vi "solar_gbl Read Config.vi"(8 "error in (no error)":errorcluster, 10 "Name in":string, 11 "SOLAR in":T1) -> (0 "error out":errorcluster, 1 "Targets":string[][](array[string]), 2 "Name out":string, 3 "SOLAR out":T1)   [LabVIEW 2018]
doc: "This loads the default application settings from the solar.ini configuration file. The 'AppSetups' define the different application configuration sections that can override any default configuration keys. If the override key is not defined, this uses the default SOLAR applications settings. By default, the directories are located relative to the application executable."
uses:
  solar_ctl SOLAR Global.ctl
  solar_ctl Target Global.ctl
  voyager/solar_voy_ctl Voyager Refnum.ctl
  qtimer/solar_qtimer_ctl Refnum.ctl
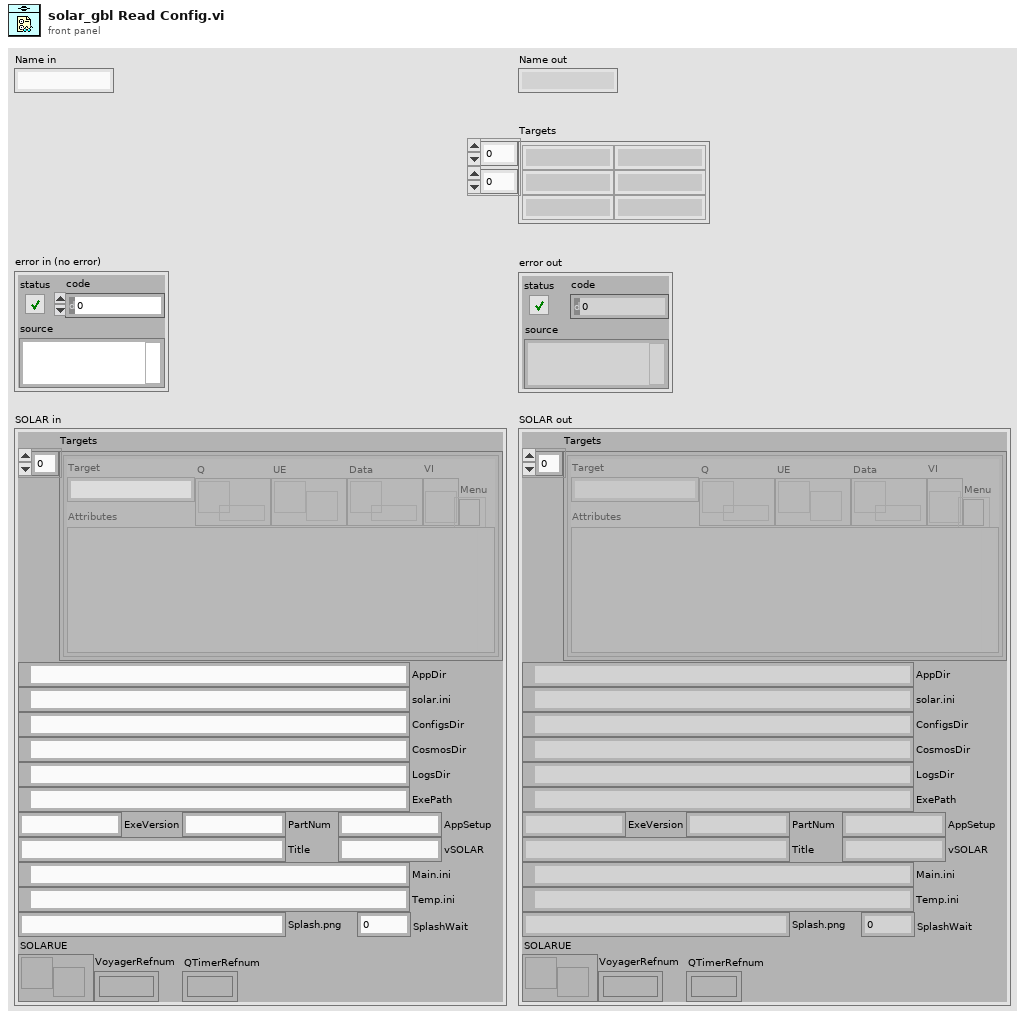
[diagram p1: front panel]
types:
  T1 = typedef "solar_ctl SOLAR Global.ctl" = cluster{"Targets":T2[], "AppDir":path, "solar.ini":path, "ConfigsDir":path, "CosmosDir":path, "LogsDir":path, "ExePath":path, "ExeVersion":string, "PartNum":string, "AppSetup":string, "Title":string, "Main.ini":path, "Temp.ini":path, "vSOLAR":string, "Splash.png":string, "SplashWait":i32, "SOLARUE":refnum<user-event>, "VoyagerRefnum":T3, "QTimerRefnum":T4}
  T2 = typedef "solar_ctl Target Global.ctl" = cluster{"Target":string, "Q":refnum<queue>, "UE":refnum<user-event>, "VI":refnum<vi>, "Menu":refnum<k9>, "Data":refnum<data-value>, "Attributes":variant}
  T3 = typedef "solar_voy_ctl Voyager Refnum.ctl" = refnum<k1>
  T4 = typedef "solar_qtimer_ctl Refnum.ctl" = refnum<k1>
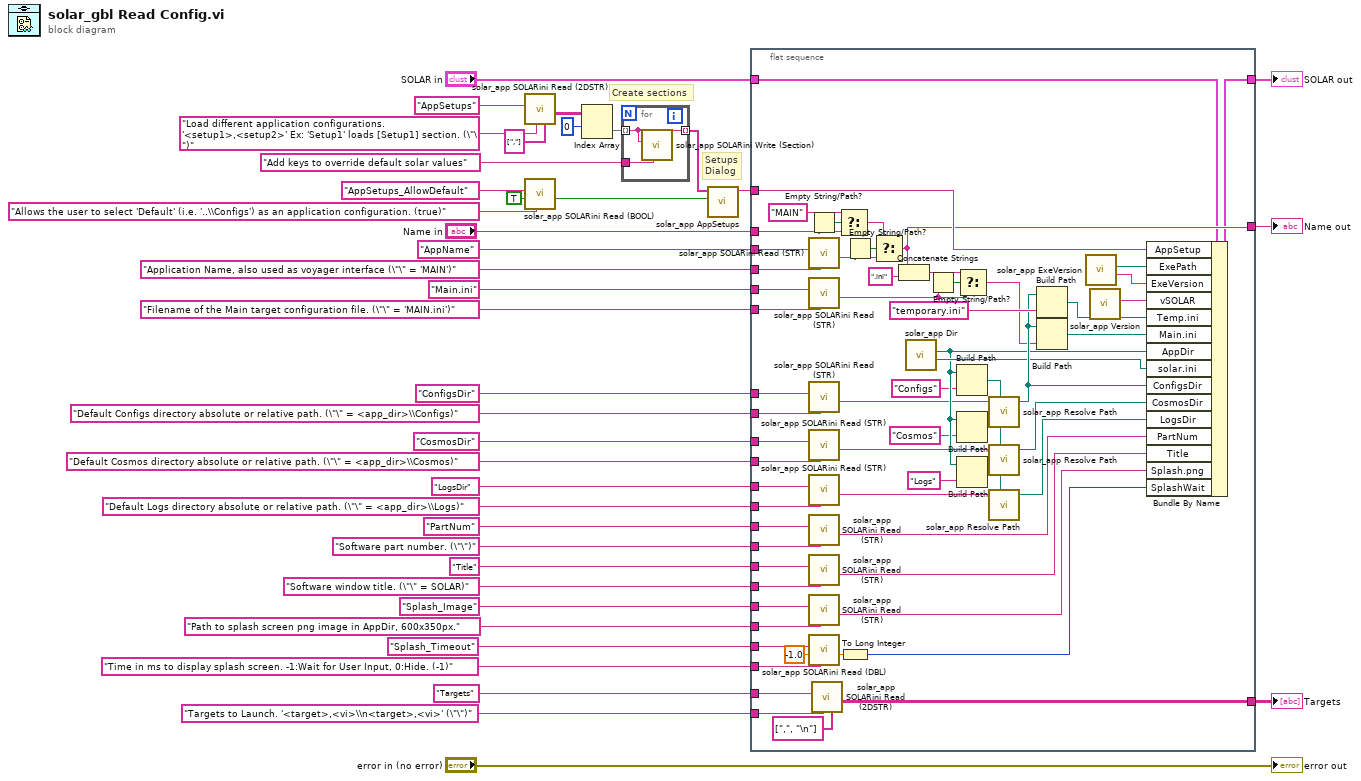
[diagram p0: block diagram]
diagram:
  # "Create sections"
  # "Setups\nDialog"
  n1 = call "solar_app SOLARini Read (2DSTR).vi"("Delimiters (1D,2D)"=string[] [","], "Comment (Create only)"="Load different application configurations. '<setup1>,<setup2>' Ex: 'Setup1' loads [Setup1] section. (\"\")", "Key"="AppSetups") -> ("Value (STR) out"=w36:string[][])  [unwired: 7 in, 1 out]
  n2 = call "solar_app SOLARini Read (BOOL).vi"("Comment (Create only)"="Allows the user to select 'Default' (i.e. '..\\Configs') as an application configuration. (true)", "Default Value (BOOL)"=TRUE, "Key"="AppSetups_AllowDefault") -> ("Value (BOOL) out"=w37:bool)  [unwired: 7 in, 1 out]
  n3 = Index Array(array=w36, index (row)=0) -> (element=w3:string[])  [unwired: 1 in]
  n4 = for {
    tunnel: w3 -> [w41] mode=indexing
    tunnel: [w41] -> w1 mode=indexing
    tunnel: "Add keys to override default solar values" ("Comment (Create only)") -> [w40]
    n5 = call "solar_app SOLARini Write (Section).vi"("Comment (Create only)"=w40, "Section"=w41) -> ()  [unwired: 9 in, 1 out]
  }
  n6 = call "solar_app AppSetups.vi"("AppSetups_AllowDefault"=w37, "AppSetups"=w1) -> ("Setup"=w39:string)  [unwired: 9 in]
  n7 = flat-sequence {
    tunnel: w39 -> [w103]
    tunnel: "Name in" -> [w67]
    tunnel: [w66] -> w32
    tunnel: "Default Configs directory absolute or relative path. (\"\" = <app_dir>\\Configs)" ("Comment (Create only)") -> [w65]
    tunnel: "Default Cosmos directory absolute or relative path. (\"\" = <app_dir>\\Cosmos)" ("Comment (Create only)") -> [w64]
    tunnel: "Default Logs directory absolute or relative path. (\"\" = <app_dir>\\Logs)" ("Comment (Create only)") -> [w63]
    tunnel: "Software part number. (\"\")" ("Comment (Create only)") -> [w62]
    tunnel: "Software window title. (\"\" = SOLAR)" ("Comment (Create only)") -> [w61]
    tunnel: "Filename of the Main target configuration file. (\"\" = 'MAIN.ini')" ("Comment (Create only)") -> [w60]
    tunnel: "Time in ms to display splash screen. -1:Wait for User Input, 0:Hide. (-1)" ("Comment (Create only)") -> [w59]
    tunnel: "Application Name, also used as voyager interface (\"\" = 'MAIN')" ("Comment (Create only)") -> [w58]
    tunnel: "Targets to Launch. '<target>,<vi>\\n<target>,<vi>' (\"\")" ("Comment (Create only)") -> [w57]
    tunnel: "Path to splash screen png image in AppDir, 600x350px." ("Comment (Create only)") -> [w56]
    tunnel: "Targets" ("Key") -> [w55]
    tunnel: "Splash_Image" ("Key") -> [w54]
    tunnel: "Splash_Timeout" ("Key") -> [w53]
    tunnel: "AppName" ("Key") -> [w52]
    tunnel: "Main.ini" ("Key") -> [w51]
    tunnel: "Title" ("Key") -> [w50]
    tunnel: "PartNum" ("Key") -> [w49]
    tunnel: "LogsDir" ("Key") -> [w48]
    tunnel: "CosmosDir" ("Key") -> [w47]
    tunnel: "ConfigsDir" ("Key") -> [w46]
    tunnel: "SOLAR in" -> [w45]
    tunnel: [w44] -> w6
    tunnel: [w43] -> w5
    frame #0 {
      n8 = Empty String/Path?(string/path=w67) -> (empty?=w101:bool)
      n9 = call "solar_app SOLARini Read (STR).vi"("Comment (Create only)"=w58, "Key"=w52) -> ("Value (STR) out"=w84:string)  [unwired: 8 in, 1 out]
      n10 = call "solar_app SOLARini Read (STR).vi"("Comment (Create only)"=w60, "Key"=w51) -> ("Value (STR) out"=w87:string)  [unwired: 8 in, 1 out]
      n11 = call "solar_app SOLARini Read (STR).vi"("Comment (Create only)"=w65, "Key"=w46) -> ("Value (STR) out"=w69:string)  [unwired: 8 in, 1 out]
      n12 = call "solar_app SOLARini Read (STR).vi"("Comment (Create only)"=w64, "Key"=w47) -> ("Value (STR) out"=w74:string)  [unwired: 8 in, 1 out]
      n13 = call "solar_app SOLARini Read (STR).vi"("Comment (Create only)"=w63, "Key"=w48) -> ("Value (STR) out"=w77:string)  [unwired: 8 in, 1 out]
      n14 = call "solar_app SOLARini Read (STR).vi"("Comment (Create only)"=w62, "Key"=w49) -> ("Value (STR) out"=w82:string)  [unwired: 8 in, 1 out]
      n15 = call "solar_app SOLARini Read (STR).vi"("Comment (Create only)"=w61, "Key"=w50) -> ("Value (STR) out"=w83:string)  [unwired: 8 in, 1 out]
      n16 = call "solar_app SOLARini Read (STR).vi"("Comment (Create only)"=w56, "Key"=w54) -> ("Value (STR) out"=w98:string)  [unwired: 8 in, 1 out]
      n17 = call "solar_app SOLARini Read (DBL).vi"("Comment (Create only)"=w59, "Default Value (DBL)"=-1.0, "Key"=w53) -> ("Value (DBL) out"=w99:dbl)  [unwired: 7 in, 1 out]
      n18 = call "solar_app SOLARini Read (2DSTR).vi"("Delimiters (1D,2D)"=string[] [",", "\n"], "Comment (Create only)"=w57, "Key"=w55) -> ("Value (STR) out"=w43:string[][])  [unwired: 7 in, 1 out]
      n19 = Select(t="MAIN", s=w101, f=w67) -> (s? t:f=w102:string)
      n20 = To Long Integer(number=w99) -> (32bit integer=w42:i32)
      n21 = Empty String/Path?(string/path=w84) -> (empty?=w85:bool)
      n22 = Select(t=w102, s=w85, f=w84) -> (s? t:f=w66:string)
      n23 = Concatenate Strings(w66, ".ini" ("string")) -> (w89:string)
      n24 = call "solar_app Dir.vi"() -> ("solar.ini"=w79:path, "AppDir"=w78:path)  [unwired: 9 in, 1 out]
      n25 = Empty String/Path?(string/path=w87) -> (empty?=w86:bool)
      n26 = Build Path(base path=w78, name or relative path="Configs") -> (appended path=w70:path)
      n27 = Build Path(base path=w78, name or relative path="Cosmos") -> (appended path=w73:path)
      n28 = Build Path(base path=w78, name or relative path="Logs") -> (appended path=w75:path)
      n29 = Select(t=w89, s=w86, f=w87) -> (s? t:f=w90:string)
      n30 = call "solar_app Resolve Path.vi"("Path to Resolve (\"\"=default Path)"=w69, "default Path"=w70) -> ("Resolved Path"=w92:path)  [unwired: 6 in, 1 out]
      n31 = call "solar_app Resolve Path.vi"("Path to Resolve (\"\"=default Path)"=w74, "default Path"=w73) -> ("Resolved Path"=w80:path)  [unwired: 6 in, 1 out]
      n32 = call "solar_app Resolve Path.vi"("Path to Resolve (\"\"=default Path)"=w77, "default Path"=w75) -> ("Resolved Path"=w81:path)  [unwired: 6 in, 1 out]
      n33 = Build Path(base path=w92, name or relative path="temporary.ini") -> (appended path=w104:path)
      n34 = Build Path(base path=w92, name or relative path=w90) -> (appended path=w91:path)
      n35 = call "solar_app ExeVersion.vi"() -> ("ExeVersion"=w95:string, "ExePath"=w94:path)  [unwired: 9 in, 1 out]
      n36 = call "solar_app Version.vi"() -> ("SOLAR Version"=w96:string)  [unwired: 11 in]
      n37 = Bundle By Name(cluster=w45, "AppSetup"=w103, "ExePath"=w94, "ExeVersion"=w95, "vSOLAR"=w96, "Temp.ini"=w104, "Main.ini"=w91, "AppDir"=w78, "solar.ini"=w79, "ConfigsDir"=w92, "CosmosDir"=w80, "LogsDir"=w81, "PartNum"=w82, "Title"=w83, "Splash.png"=w98, "SplashWait"=w42) -> (w44:T1)
    }
  }
  "Name out" <- w32
  "SOLAR out" <- w6
  "Targets" <- w5
  "error out" <- "error in (no error)"
